vi "test-Mecanum-Odometry-Test1.vi"() -> (3 "All tests passed":bool)   [LabVIEW 2019]
uses:
  <vilib>/Rock Robotics/WPI/ThirdParty/JAS_Junk/TrajLib/Rotation2d_CreateAngle.vi
  <vilib>/Rock Robotics/WPI/ThirdParty/JAS_Junk/TrajLib/Trajectory_Library.lvlib
panel:
  out "Test 4":bool
  out "Test 3":bool
  out "Test 2":bool
  out "Test 1":bool
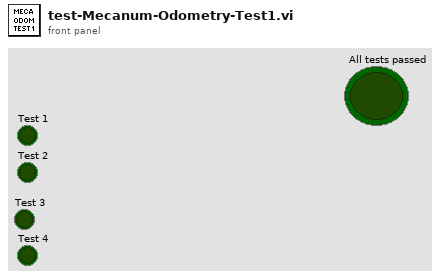
[diagram p1: front panel]
types:
  T1 = typedef "Trajectory_Library.lvlib/MECA_WHEEL_POSITIONS.ctl" = cluster{"FrontLeft":dbl, "FrontRight":dbl, "RearLeft":dbl, "RearRight":dbl, "X":bool}
  T2 = typedef "Trajectory_Library.lvlib/ROTATION2D.ctl" = cluster{"VALUE":dbl, "COS":dbl, "SIN":dbl}
  T3 = typedef "Trajectory_Library.lvlib/POSE2D.ctl" = cluster{"TRANSLATION":T4, "ROTATION":T2}
  T4 = typedef "Trajectory_Library.lvlib/TRANSLATION2D.ctl" = cluster{"X":dbl, "Y":dbl}
  T5 = typedef "Trajectory_Library.lvlib/MECA_DRIVE_KINEMATICS.ctl" = cluster{"FrontLeft":T4, "FrontRight":T4, "RearLeft":T4, "RearRight":T4, "InverseKinematics":T6, "ForwardKinematics":T6, "PrevCoR":T4}
  T6 = typedef "NI_Matrix.lvlib/RealMatrix.ctl" = dbl[][]
  T7 = typedef "Trajectory_Library.lvlib/MECA_DRIVE_ODOMETRY.ctl" = cluster{"POSE":T3, "GyroOffset":T2, "PreviousAngle":T2, "Kinematics":T5, "PreviousWheelPositions":T1}
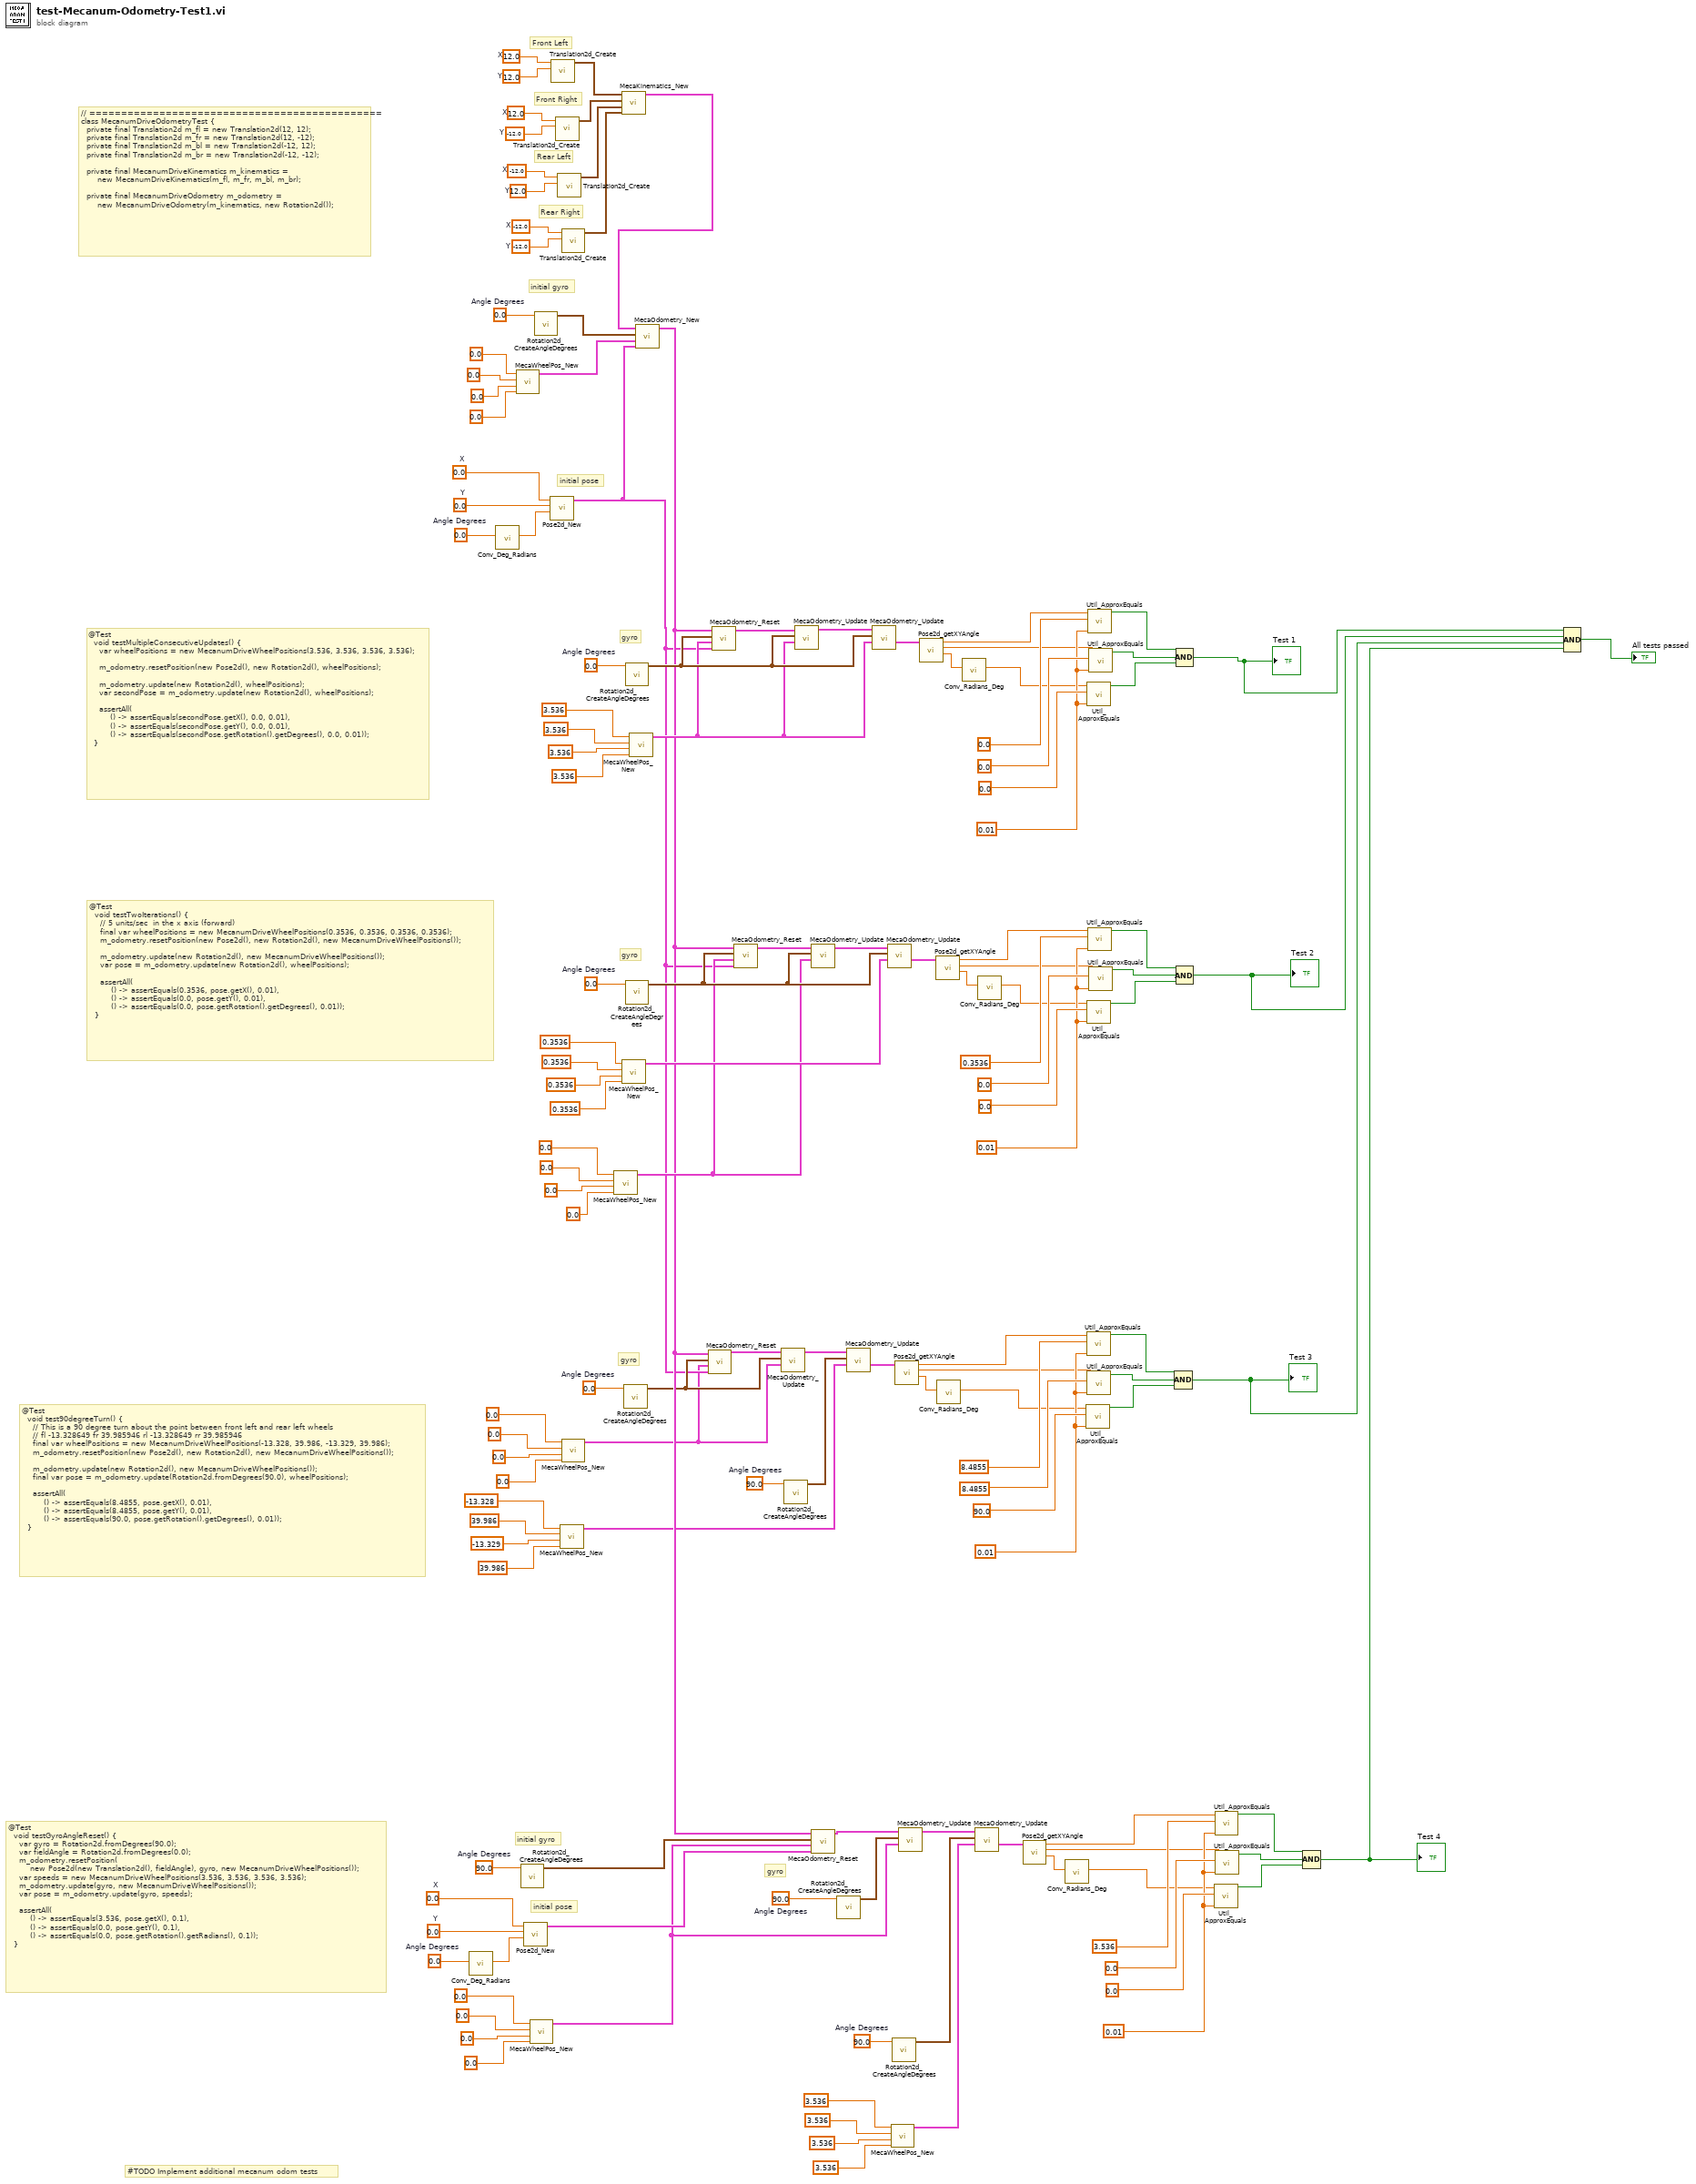
[diagram p0: block diagram]
diagram:
  w42 = 90.0  # Angle Degrees
  w46 = 0.0  # X
  w45 = 0.0  # Y
  w43 = 0.0  # Angle Degrees
  w49 = 90.0  # Angle Degrees
  w56 = 90.0  # Angle Degrees
  w58 = 0.01 ("Tolerance")
  w67 = 90.0  # Angle Degrees
  w77 = 0.0  # Angle Degrees
  w83 = 0.01 ("Tolerance")
  w96 = 0.0  # Angle Degrees
  w98 = 0.01 ("Tolerance")
  w110 = 0.0  # Angle Degrees
  w116 = 0.0  # Angle Degrees
  w120 = 0.0  # X
  w119 = 0.0  # Y
  w117 = 0.0  # Angle Degrees
  w121 = 0.01 ("Tolerance")
  w136 = -12.0  # X
  w135 = -12.0  # Y
  w134 = -12.0  # X
  w133 = 12.0  # Y
  w132 = 12.0  # X
  w131 = -12.0  # Y
  w130 = 12.0  # X
  w129 = 12.0  # Y
  # "@Test\n  void testGyroAngleReset() {\n    var gyro = Rotation2d.fromDegrees(90.0);\n    var fieldAngle = Rotation2d.fromDegrees(0.0);\n    m_odometry.resetPosition(\n        new Pose2d(new Translation2d(), fieldAngle), gyro, new MecanumDriveWheelPositions());\n    var speeds = new MecanumDriveWheelPositions(3.536, 3.536, 3.536, 3.536);\n    m_odometry.update(gyro, new MecanumDriveWheelPositions());\n    var pose = m_odometry.update(gyro, speeds);\n\n    assertAll(\n        () -> assertEquals(3.536, pose.getX(), 0.1),\n        () -> assertEquals(0.0, pose.getY(), 0.1),\n        () -> assertEquals(0.0, pose.getRotation().getRadians(), 0.1));\n  }"
  # "#TODO Implement additional mecanum odom tests"
  # "@Test\n  void test90degreeTurn() {\n    // This is a 90 degree turn about the point between front left and rear left wheels\n    // fl -13.328649 fr 39.985946 rl -13.328649 rr 39.985946\n    final var wheelPositions = new MecanumDriveWheelPositions(-13.328, 39.986, -13.329, 39.986);\n    m_odometry.resetPosition(new Pose2d(), new Rotation2d(), new MecanumDriveWheelPositions());\n\n    m_odometry.update(new Rotation2d(), new MecanumDriveWheelPositions());\n    final var pose = m_odometry.update(Rotation2d.fromDegrees(90.0), wheelPositions);\n\n    assertAll(\n        () -> assertEquals(8.4855, pose.getX(), 0.01),\n        () -> assertEquals(8.4855, pose.getY(), 0.01),\n        () -> assertEquals(90.0, pose.getRotation().getDegrees(), 0.01));\n  }"
  # "@Test\n  void testTwoIterations() {\n    // 5 units/sec  in the x axis (forward)\n    final var wheelPositions = new MecanumDriveWheelPositions(0.3536, 0.3536, 0.3536, 0.3536);\n    m_odometry.resetPosition(new Pose2d(), new Rotation2d(), new MecanumDriveWheelPositions());\n\n    m_odometry.update(new Rotation2d(), new MecanumDriveWheelPositions());\n    var pose = m_odometry.update(new Rotation2d(), wheelPositions);\n\n    assertAll(\n        () -> assertEquals(0.3536, pose.getX(), 0.01),\n        () -> assertEquals(0.0, pose.getY(), 0.01),\n        () -> assertEquals(0.0, pose.getRotation().getDegrees(), 0.01));\n  }"
  # "@Test\n  void testMultipleConsecutiveUpdates() {\n    var wheelPositions = new MecanumDriveWheelPositions(3.536, 3.536, 3.536, 3.536);\n\n    m_odometry.resetPosition(new Pose2d(), new Rotation2d(), wheelPositions);\n\n    m_odometry.update(new Rotation2d(), wheelPositions);\n    var secondPose = m_odometry.update(new Rotation2d(), wheelPositions);\n\n    assertAll(\n        () -> assertEquals(secondPose.getX(), 0.0, 0.01),\n        () -> assertEquals(secondPose.getY(), 0.0, 0.01),\n        () -> assertEquals(secondPose.getRotation().getDegrees(), 0.0, 0.01));\n  }"
  # "initial gyro"
  # "initial pose"
  # "gyro"
  # "gyro"
  # "gyro"
  # "gyro"
  # "initial gyro"
  # "initial pose"
  # "Rear Right"
  # "Rear Left"
  # "Front Right"
  # "Front Left"
  # "// ==============================================\nclass MecanumDriveOdometryTest {\n  private final Translation2d m_fl = new Translation2d(12, 12);\n  private final Translation2d m_fr = new Translation2d(12, -12);\n  private final Translation2d m_bl = new Translation2d(-12, 12);\n  private final Translation2d m_br = new Translation2d(-12, -12);\n\n  private final MecanumDriveKinematics m_kinematics =\n      new MecanumDriveKinematics(m_fl, m_fr, m_bl, m_br);\n\n  private final MecanumDriveOdometry m_odometry =\n      new MecanumDriveOdometry(m_kinematics, new Rotation2d());"
  n1 = call <vilib>:"Conv_Deg_Radians.vi"("Degress"=w43) -> ("Radians"=w44:dbl)  [unwired: 10 in]
  n2 = call <vilib>:"Conv_Deg_Radians.vi"("Degress"=w117) -> ("Radians"=w118:dbl)  [unwired: 10 in]
  n3 = call <vilib>:"MecaWheelPos_New.vi"("RearRightPosition"=0.0, "RearLeftPosition"=0.0, "FrontRightPosition"=0.0, "FrontLeftPosition"=0.0) -> ("MECA_WHEEL_POSITIONS"=w33:T1)  [unwired: 7 in]
  n4 = call <vilib>:"Rotation2d_CreateAngleDegrees.vi"("Angle_Degrees"=w42) -> ("ROTATION"=w41:T2)  [unwired: 10 in]
  n5 = call <vilib>:"Pose2d_New.vi"("Heading"=w44, "Y"=w45, "X"=w46) -> ("out POSe"=w11:T3)  [unwired: 8 in]
  n6 = call <vilib>:"MecaWheelPos_New.vi"("RearRightPosition"=0.0 ("RearRightSpeed"), "RearLeftPosition"=0.0 ("RearLeftSpeed"), "FrontRightPosition"=0.0 ("FrontRightSpeed"), "FrontLeftPosition"=0.0 ("FrontLeftSpeed")) -> ("MECA_WHEEL_POSITIONS"=w2:T1)  [unwired: 7 in]
  n7 = call <vilib>:"Rotation2d_CreateAngleDegrees.vi"("Angle_Degrees"=w116) -> ("ROTATION"=w39:T2)  [unwired: 10 in]
  n8 = call <vilib>:"Pose2d_New.vi"("Heading"=w118, "Y"=w119, "X"=w120) -> ("out POSe"=w14:T3)  [unwired: 8 in]
  n9 = call <vilib>:"Translation2d_Create.vi"("Y"=w129, "X"=w130) -> ("TRANSLATION"=w137:T4)  [unwired: 9 in]
  n10 = call <vilib>:"Translation2d_Create.vi"("Y"=w131, "X"=w132) -> ("TRANSLATION"=w138:T4)  [unwired: 9 in]
  n11 = call <vilib>:"Translation2d_Create.vi"("Y"=w133, "X"=w134) -> ("TRANSLATION"=w139:T4)  [unwired: 9 in]
  n12 = call <vilib>:"MecaWheelPos_New.vi"("RearRightPosition"=39.986 ("RearRightSpeed"), "RearLeftPosition"=-13.329 ("RearLeftSpeed"), "FrontRightPosition"=39.986 ("FrontRightSpeed"), "FrontLeftPosition"=-13.328 ("FrontLeftSpeed")) -> ("MECA_WHEEL_POSITIONS"=w12:T1)  [unwired: 7 in]
  n13 = call <vilib>:"Translation2d_Create.vi"("Y"=w135, "X"=w136) -> ("TRANSLATION"=w140:T4)  [unwired: 9 in]
  n14 = call <vilib>:"MecaWheelPos_New.vi"("RearRightPosition"=0.0 ("RearRightSpeed"), "RearLeftPosition"=0.0 ("RearLeftSpeed"), "FrontRightPosition"=0.0 ("FrontRightSpeed"), "FrontLeftPosition"=0.0 ("FrontLeftSpeed")) -> ("MECA_WHEEL_POSITIONS"=w13:T1)  [unwired: 7 in]
  n15 = call <vilib>:"MecaWheelPos_New.vi"("RearRightPosition"=0.0 ("RearRightSpeed"), "RearLeftPosition"=0.0 ("RearLeftSpeed"), "FrontRightPosition"=0.0 ("FrontRightSpeed"), "FrontLeftPosition"=0.0 ("FrontLeftSpeed")) -> ("MECA_WHEEL_POSITIONS"=w18:T1)  [unwired: 7 in]
  n16 = call <vilib>:"MecaKinematics_New.vi"("RearRight"=w140, "RearLeft"=w139, "FrontRight"=w138, "FrontLeft"=w137) -> ("MECA_DRIVE_KINEMATICS"=w38:T5)  [unwired: 7 in]
  n17 = call <vilib>:"MecaWheelPos_New.vi"("RearRightPosition"=0.3536 ("RearRightSpeed"), "RearLeftPosition"=0.3536 ("RearLeftSpeed"), "FrontRightPosition"=0.3536 ("FrontRightSpeed"), "FrontLeftPosition"=0.3536 ("FrontLeftSpeed")) -> ("MECA_WHEEL_POSITIONS"=w19:T1)  [unwired: 7 in]
  n18 = call <vilib>:"Rotation2d_CreateAngleDegrees.vi"("Angle_Degrees"=w77) -> ("ROTATION"=w15:T2)  [unwired: 10 in]
  n19 = call <vilib>:"Rotation2d_CreateAngleDegrees.vi"("Angle_Degrees"=w110) -> ("ROTATION"=w23:T2)  [unwired: 10 in]
  n20 = call <vilib>:"Rotation2d_CreateAngleDegrees.vi"("Angle_Degrees"=w96) -> ("ROTATION"=w20:T2)  [unwired: 10 in]
  n21 = call <vilib>:"MecaWheelPos_New.vi"("RearRightPosition"=3.536 ("RearRightSpeed"), "RearLeftPosition"=3.536 ("RearLeftSpeed"), "FrontRightPosition"=3.536 ("FrontRightSpeed"), "FrontLeftPosition"=3.536 ("FrontLeftSpeed")) -> ("MECA_WHEEL_POSITIONS"=w21:T1)  [unwired: 7 in]
  n22 = call <vilib>:"MecaOdometry_New.vi"("Initial Pose2d"=w14, "wheelPositions"=w33, "GyroOffset"=w39, "Mecanum Kinematics"=w38) -> ("MECA_DRIVE_ODOMETRY"=w17:T7)  [unwired: 7 in]
  n23 = call <vilib>:"MecaOdometry_Reset.vi"("POSE"=w14, "WheelPositions"=w13, "GyroOffset"=w15, "in MECA_DRIVE_ODOMETRY"=w17) -> ("out MECA_DRIVE_ODOMETRY"=w16:T7)  [unwired: 7 in]
  n24 = call <vilib>:"MecaOdometry_Reset.vi"("POSE"=w14, "WheelPositions"=w21, "GyroOffset"=w23, "in MECA_DRIVE_ODOMETRY"=w17) -> ("out MECA_DRIVE_ODOMETRY"=w24:T7)  [unwired: 7 in]
  n25 = call <vilib>:"MecaOdometry_Reset.vi"("POSE"=w14, "WheelPositions"=w18, "GyroOffset"=w20, "in MECA_DRIVE_ODOMETRY"=w17) -> ("out MECA_DRIVE_ODOMETRY"=w22:T7)  [unwired: 7 in]
  n26 = call <vilib>:"MecaOdometry_Update.vi"("WheelPosition"=w13, "GyroAngle"=w15, "in MECA_DRIVE_ODOMETRY"=w16) -> ("out MECA_DRIVE_ODOMETRY"=w78:T7)  [unwired: 7 in, 1 out]
  n27 = call <vilib>:"Rotation2d_CreateAngleDegrees.vi"("Angle_Degrees"=w67) -> ("ROTATION"=w66:T2)  [unwired: 10 in]
  n28 = call <vilib>:"MecaOdometry_Update.vi"("WheelPosition"=w21, "GyroAngle"=w23, "in MECA_DRIVE_ODOMETRY"=w24) -> ("out MECA_DRIVE_ODOMETRY"=w111:T7)  [unwired: 7 in, 1 out]
  n29 = call <vilib>:"MecaOdometry_Update.vi"("WheelPosition"=w18, "GyroAngle"=w20, "in MECA_DRIVE_ODOMETRY"=w22) -> ("out MECA_DRIVE_ODOMETRY"=w97:T7)  [unwired: 7 in, 1 out]
  n30 = call <vilib>:"MecaOdometry_Reset.vi"("POSE"=w11, "WheelPositions"=w2, "GyroOffset"=w41, "in MECA_DRIVE_ODOMETRY"=w17) -> ("out MECA_DRIVE_ODOMETRY"=w47:T7)  [unwired: 7 in]
  n31 = call <vilib>:"Rotation2d_CreateAngleDegrees.vi"("Angle_Degrees"=w56) -> ("ROTATION"=w55:T2)  [unwired: 10 in]
  n32 = call <vilib>:"MecaOdometry_Update.vi"("WheelPosition"=w12, "GyroAngle"=w66, "in MECA_DRIVE_ODOMETRY"=w78) -> ("POSE"=w76:T3)  [unwired: 7 in, 1 out]
  n33 = call <vilib>:"MecaOdometry_Update.vi"("WheelPosition"=w21, "GyroAngle"=w23, "in MECA_DRIVE_ODOMETRY"=w111) -> ("POSE"=w109:T3)  [unwired: 7 in, 1 out]
  n34 = call <vilib>:"MecaOdometry_Update.vi"("WheelPosition"=w19, "GyroAngle"=w20, "in MECA_DRIVE_ODOMETRY"=w97) -> ("POSE"=w95:T3)  [unwired: 7 in, 1 out]
  n35 = call <vilib>:"MecaWheelPos_New.vi"("RearRightPosition"=3.536 ("RearRightSpeed"), "RearLeftPosition"=3.536 ("RearLeftSpeed"), "FrontRightPosition"=3.536 ("FrontRightSpeed"), "FrontLeftPosition"=3.536 ("FrontLeftSpeed")) -> ("MECA_WHEEL_POSITIONS"=w1:T1)  [unwired: 7 in]
  n36 = call <vilib>:"Rotation2d_CreateAngleDegrees.vi"("Angle_Degrees"=w49) -> ("ROTATION"=w48:T2)  [unwired: 10 in]
  n37 = call <vilib>:"Pose2d_getXYAngle.vi"("in POSE"=w76) -> ("Angle"=w75:dbl, "Y"=w73:dbl, "X"=w74:dbl)  [unwired: 8 in]
  n38 = call <vilib>:"MecaOdometry_Update.vi"("WheelPosition"=w2, "GyroAngle"=w55, "in MECA_DRIVE_ODOMETRY"=w47) -> ("out MECA_DRIVE_ODOMETRY"=w57:T7)  [unwired: 7 in, 1 out]
  n39 = call <vilib>:"Pose2d_getXYAngle.vi"("in POSE"=w109) -> ("Angle"=w108:dbl, "Y"=w106:dbl, "X"=w107:dbl)  [unwired: 8 in]
  n40 = call <vilib>:"Pose2d_getXYAngle.vi"("in POSE"=w95) -> ("Angle"=w94:dbl, "Y"=w92:dbl, "X"=w93:dbl)  [unwired: 8 in]
  n41 = call <vilib>:"Conv_Radians_Deg.vi"("Radians"=w75) -> ("Degrees"=w72:dbl)  [unwired: 10 in]
  n42 = call <vilib>:"Conv_Radians_Deg.vi"("Radians"=w108) -> ("Degrees"=w105:dbl)  [unwired: 10 in]
  n43 = call <vilib>:"MecaOdometry_Update.vi"("WheelPosition"=w1, "GyroAngle"=w48, "in MECA_DRIVE_ODOMETRY"=w57) -> ("POSE"=w54:T3)  [unwired: 7 in, 1 out]
  n44 = call <vilib>:"Conv_Radians_Deg.vi"("Radians"=w94) -> ("Degrees"=w91:dbl)  [unwired: 10 in]
  n45 = call <vilib>:"Pose2d_getXYAngle.vi"("in POSE"=w54) -> ("Angle"=w53:dbl, "Y"=w51:dbl, "X"=w52:dbl)  [unwired: 8 in]
  n46 = call <vilib>:"Conv_Radians_Deg.vi"("Radians"=w53) -> ("Degrees"=w50:dbl)  [unwired: 10 in]
  n47 = call <vilib>:"Util_ApproxEquals.vi"("Tolerance"=w83, "Value 2"=90.0, "Value 1"=w72) -> ("ApproxEquals"=w84:bool)  [unwired: 8 in]
  n48 = call <vilib>:"Util_ApproxEquals.vi"("Tolerance"=w83, "Value 2"=8.4855, "Value 1"=w74) -> ("ApproxEquals"=w86:bool)  [unwired: 8 in]
  n49 = call <vilib>:"Util_ApproxEquals.vi"("Tolerance"=w121, "Value 2"=0.0, "Value 1"=w105) -> ("ApproxEquals"=w123:bool)  [unwired: 8 in]
  n50 = call <vilib>:"Util_ApproxEquals.vi"("Tolerance"=w98, "Value 2"=0.0, "Value 1"=w91) -> ("ApproxEquals"=w99:bool)  [unwired: 8 in]
  n51 = call <vilib>:"Util_ApproxEquals.vi"("Tolerance"=w83, "Value 2"=8.4855, "Value 1"=w73) -> ("ApproxEquals"=w85:bool)  [unwired: 8 in]
  n52 = call <vilib>:"Util_ApproxEquals.vi"("Tolerance"=w121, "Value 2"=0.0, "Value 1"=w107) -> ("ApproxEquals"=w125:bool)  [unwired: 8 in]
  n53 = call <vilib>:"Util_ApproxEquals.vi"("Tolerance"=w98, "Value 2"=0.3536, "Value 1"=w93) -> ("ApproxEquals"=w101:bool)  [unwired: 8 in]
  n54 = call <vilib>:"Util_ApproxEquals.vi"("Tolerance"=w121, "Value 2"=0.0, "Value 1"=w106) -> ("ApproxEquals"=w124:bool)  [unwired: 8 in]
  n55 = call <vilib>:"Util_ApproxEquals.vi"("Tolerance"=w98, "Value 2"=0.0, "Value 1"=w92) -> ("ApproxEquals"=w100:bool)  [unwired: 8 in]
  n56 = Compound Arithmetic op=AND(w86, w85, w84) -> (w65:bool)
  "Test 3" <- w65
  n57 = Compound Arithmetic op=AND(w125, w124, w123) -> (w122:bool)
  "Test 1" <- w122
  n58 = Compound Arithmetic op=AND(w101, w100, w99) -> (w90:bool)
  "Test 2" <- w90
  n59 = call <vilib>:"Util_ApproxEquals.vi"("Tolerance"=w58, "Value 2"=0.0, "Value 1"=w50) -> ("ApproxEquals"=w59:bool)  [unwired: 8 in]
  n60 = call <vilib>:"Util_ApproxEquals.vi"("Tolerance"=w58, "Value 2"=3.536, "Value 1"=w52) -> ("ApproxEquals"=w61:bool)  [unwired: 8 in]
  n61 = call <vilib>:"Util_ApproxEquals.vi"("Tolerance"=w58, "Value 2"=0.0, "Value 1"=w51) -> ("ApproxEquals"=w60:bool)  [unwired: 8 in]
  n62 = Compound Arithmetic op=AND(w61, w60, w59) -> (w40:bool)
  "Test 4" <- w40
  n63 = Compound Arithmetic op=AND(w122, w90, w65, w40) -> (→"All tests passed":bool)
